vi "UHR-Fleezers Control (host) - Lorentz v3.vi"() -> ()   [LabVIEW 2014] (continued)
                            n445 = Not(x=w776) -> (.not. x?=w775:bool)
                            n446 = Compound Arithmetic op=OR(w779, "Cancel dwell", w775) -> (w778:bool)
                            n447 = node-c288() -> ()  [unwired: 1 in, 1 out]
                            n448 = Select(t=FALSE, s="Pause dwell", f=w778) -> (s? t:f=w781:bool)
                            n449 = Or(x=w781, y=w773) -> (x .or. y?=w774:bool)
                            "Dwell Time (s)" <- w772
                          }
                          n450 = node-c288(w770) -> ()  [unwired: 1 out]
                        }
                      }
                    }
                  }
                }
                frame #4 {
                  n451 = local read "Dip for Protein"() -> (w791:bool)
                  n452 = local read "Dump Beads"() -> (w788:bool)
                  n453 = local write "Cancel dwell"(FALSE ("Cancel dwell")) -> ()
                  n454 = Not(x=w791) -> (.not. x?=w792:bool)
                  n455 = Not(x="Cont. Repeat Dipping?") -> (.not. x?=w794:bool)
                  n456 = Compound Arithmetic op=OR(w792, w794, w788) -> (w790:bool)
                }
              }
            }
          }
        }
      }
      event "Profile": Value Change {
        n457 = event-data() -> ()  [unwired: 1 in, 5 out]
        n458 = flat-sequence {
          tunnel: w803 -> [w806]
          tunnel: w802 -> [w814]
          tunnel: [w808] -> w801
          tunnel: [w807] -> w800
          tunnel: [w805] -> w798
          tunnel: [w804] -> w795
          tunnel: w801 -> [w821]
          tunnel: w800 -> [w820]
          tunnel: [w818] -> w799
          tunnel: w798 -> [w819]
          tunnel: [w817] -> w797
          tunnel: [w816] -> w796
          tunnel: w795 -> [w816]
          tunnel: w799 -> [w825]
          tunnel: w797 -> [w824]
          tunnel: w796 -> [w823]
          frame #0 {
            n459 = call "Read Stage Position.vi"("error in"=w814, "VISA resource name in"=w806) -> ("Current Position"=w804:cluster{dbl, dbl, dbl}, "error out"=w807:errorcluster, "VISA resource name out"=w805:refnum<visa-resource-name>)  [unwired: 1 out]
            "Current Position" <- w804
            n460 = local write "Stage Control Serial Error"(w807) -> ()
            n461 = Unbundle(w804) -> (w811:dbl, w813:dbl, w809:dbl)
            n462 = Add(x=w813, y="Y change (mm)") -> (x+y=w810:dbl)
            n463 = Bundle(w811, w810, w809) -> (w808:cluster{dbl, dbl, dbl})  [unwired: 1 in]
          }
          frame #1 {
            # "move to new position and start saving"
            n464 = local write "Stage Moving"(TRUE ("Stage Moving")) -> ()
            n465 = local write "Start Saving"(TRUE ("Start Saving")) -> ()
            n466 = call "Set Stage Position.vi"("Position"=w821, "error in"=w820, "VISA resource name in"=w819) -> ("error out"=w817:errorcluster, "VISA resource name out"=w818:refnum<visa-resource-name>)  [unwired: 1 out]
          }
          frame #2 {
            # "go back to start"
            n467 = call "Set Stage Position.vi"("Position"=w823, "error in"=w824, "VISA resource name in"=w825) -> ()  [unwired: 3 out]
          }
          frame #3 {
            # "stop saving"
            n468 = local write "Stop Saving"(TRUE ("Stop Saving")) -> ()
            n469 = local write "Stage Moving"(FALSE ("Stage Moving")) -> ()
          }
        }
      }
      event "Move to Position 1", "Move to Position 2", "Move to Position 3", "Move to Position 4", "Move to Position 5", "Lower Ch. Cap.", "Move to Position 6": Value Change {
        n470 = event-data() -> ()  [unwired: 1 in, 5 out]
        n471 = Or(x="Move to Position 5", y="Lower Ch. Cap.") -> (x .or. y?=w832:bool)
        n472 = Build Array("Move to Position 1", "Move to Position 2", "Move to Position 3", "Move to Position 4", w832, "Move to Position 6") -> (w835:bool[])
        n473 = Boolean Array To Number(Boolean array=w835) -> (number=w834:u32)
        n474 = Logarithm Base 2(1:w834) -> (0:w833:dbl)
        n475 = flat-sequence {
          tunnel: w833 -> [w844]
          tunnel: w830 -> [w842]
          tunnel: w829 -> [w841]
          frame #0 {
            n476 = local read "Saved Stage Positions"() -> (w852:dbl[][])
            n477 = Array Subset(array=w852, index (row)=w844, length (row)=1 ("length"), index (col)=1 ("index"), length (col)=3 ("length")) -> (w849:dbl[][])
            n478 = Reshape Array(w849, 3 ("dimension size")) -> (w847:dbl[])
            n479 = Array To Cluster(array=w847) -> (cluster=w846:cluster{"[0]":dbl, "[1]":dbl, "[2]":dbl})
            n480 = call "Set Stage Position.vi"("Position"=w846, "error in"=w841, "VISA resource name in"=w842) -> ("error out"=w845:errorcluster)  [unwired: 2 out]
            n481 = local write "Stage Moving"(TRUE ("Stage Moving")) -> ()
            n482 = local write "Stage Control Serial Error"(w845) -> ()
          }
          frame #1 {
            n483 = local write "Stage Moving"(FALSE ("Stage Moving")) -> ()
            n484 = call <vilib>:"Beep.vi"() -> ()  [unwired: 3 in, 9 out]
          }
        }
      }
      event "Got Bead 1": Value Change {
        n485 = event-data() -> ()  [unwired: 1 in, 5 out]
        n486 = flat-sequence {
          tunnel: w855 -> [w857]
          tunnel: w855 -> [w861]
          frame #0 {
            n487 = for {
              N: w857 -> [_]
              n488 = property on="Pressure Up" class="Bool (strict)"("Val(Sgnl)"=TRUE) -> ()  [unwired: 2 in, 2 out]
            }
          }
          frame #1 {
          }
          frame #2 {
            n489 = Wait (ms)(milliseconds to wait=u32 1000) -> ()  [unwired: 1 out]
          }
          frame #3 {
          }
          frame #4 {
            n490 = Multiply(x=w861, y=2) -> (x*y=w860:i32)
            n491 = for {
              N: w860 -> [_]
              n492 = property on="Vent pressure" class="Bool (strict)"("Val(Sgnl)"=TRUE) -> ()  [unwired: 2 in, 2 out]
            }
          }
          frame #5 {
            n493 = for {
              N: "Number of Pulses for bead 2" -> [_]
              n494 = property on="Pressure Up" class="Bool (strict)"("Val(Sgnl)"=TRUE) -> ()  [unwired: 2 in, 2 out]
            }
          }
        }
        n495 = local read "Number of pulses For laminar flow"() -> (w855:i32)
      }
      event "Force FB Data\nScript": Value Change {
        n496 = event-data() -> ()  [unwired: 1 in, 5 out]
        n497 = flat-sequence {
          tunnel: w871 -> [w875]
          tunnel: w872 -> [w876]
          tunnel: [w876] -> w867
          tunnel: [w875] -> w866
          tunnel: w867 -> [w879]
          tunnel: w866 -> [w878]
          tunnel: ["Trap Trig Fl."] -> w868
          tunnel: [w904] -> w869
          tunnel: w868 -> [w904]
          tunnel: [w908] -> w870
          tunnel: w869 -> [w908]
          tunnel: w870 -> [w910]
          frame #0 {
            n498 = property on="Trap Delta (MHz)" class="DigNum (strict)"("Val(Sgnl)"="Trap Delta Before Moving") -> ()  [unwired: 2 in, 2 out]
          }
          frame #1 {
            n499 = local read "Saved Stage Positions"() -> (w881:dbl[][])
            n500 = property on="Trap Pos. FB Offset Factor" class="DigNum (strict)"("Val(Sgnl)"=i64 0 ("Value (Signaling)")) -> ()  [unwired: 2 in, 2 out]
            n501 = local write "FB Trap Pos Offset"(0.0 ("FB Trap Pos Offset")) -> ()
            n502 = local write "Stage Moving"(TRUE ("Stage Moving")) -> ()
            n503 = call "move to saved stage position.vi"("error in"=w878, "Stage VISA resource name in"=w879, "Position"="Stage Position To Establish FB", "Saved Stage Positions"=w881) -> ("error out"=w877:errorcluster)  [unwired: 1 out]
            n504 = local write "Stage Control Serial Error"(w877) -> ()
          }
          frame #2 {
            n505 = call <vilib>:"Beep.vi"() -> ()  [unwired: 3 in, 9 out]
            n506 = Multiply(x="Wait (s)", y=u32 1000 ("milliseconds to wait")) -> (x*y=w888:u32)
            n507 = property on="Trap Delta (MHz)" class="DigNum (strict)"("Val(Sgnl)"="Starting \nTrap Delta (MHz)") -> ()  [unwired: 2 in, 2 out]
            n508 = local write "Stage Moving"(FALSE ("Stage Moving")) -> ()
            n509 = Wait (ms)(milliseconds to wait=w888) -> ()  [unwired: 1 out]
            n510 = property on="Tab Control 2" class="TabCtl (strict)"("Val(Sgnl)"=T11."Feedback on Trap Position" ("Value (Signaling)")) -> ()  [unwired: 2 in, 2 out]
            n511 = property on="Tab Control" class="TabCtl (strict)"("Val(Sgnl)"=T41."Trap Control (RF)" ("Value (Signaling)")) -> ()  [unwired: 2 in, 2 out]
          }
          frame #3 {
            n512 = property on="Set Reading to\nSetpoint" class="Bool (strict)"("Val(Sgnl)"=TRUE ("Value (Signaling)")) -> ()  [unwired: 2 in, 2 out]
            n513 = Wait (ms)(milliseconds to wait=u32 500) -> ()  [unwired: 1 out]
          }
          frame #4 {
            n514 = property on="Trap Pos. FB ON" class="Bool (strict)"("Val(Sgnl)"=TRUE ("Value (Signaling)")) -> ()  [unwired: 2 in, 2 out]
            n515 = Wait (ms)(milliseconds to wait=u32 250) -> ()  [unwired: 1 out]
          }
          frame #5 {
            n516 = case shown="False" "Trap Trig Fl." {
              frame False {
                n517 = case shown="True" "Green ON after FB ON?" {
                  selector: "Green ON after FB ON?" -> [_ w903]
                  frame False {
                  }
                  frame True {
                    n518 = property on="Green Laser ON" class="Bool (strict)"("Val(Sgnl)"=w903) -> ()  [unwired: 2 in, 2 out]
                  }
                }
              }
              frame True {
              }
            }
            n519 = case shown="True" "Remove Action Offset" {
              tunnel: TRUE ("Value (Signaling)") -> [w900 w901]
              frame False {
                n520 = property on="Remove Unwinding Offset" class="Bool (strict)"("Val(Sgnl)"=w900) -> ()  [unwired: 2 in, 2 out]
              }
              frame True {
                n521 = property on="Remove Action Offset" class="Bool (strict)"("Val(Sgnl)"=w901) -> ()  [unwired: 2 in, 2 out]
              }
            }
            n522 = Wait (ms)(milliseconds to wait=u32 250) -> ()  [unwired: 1 out]
          }
          frame #6 {
            n523 = property on="Start Saving" class="Bool (strict)"("Val(Sgnl)"=TRUE ("Value (Signaling)")) -> ()  [unwired: 2 in, 2 out]
            n524 = Wait (ms)(milliseconds to wait=u32 5000) -> ()  [unwired: 1 out]
          }
          frame #7 {
            w907 = TRUE ("Value (Signaling)")
            n525 = property on="Rem fb disp offset" class="Bool (strict)"("Val(Sgnl)"=w907) -> ()  [unwired: 2 in, 2 out]
            n526 = property on="Remove Offset" class="Bool (strict)"("Val(Sgnl)"=w907) -> ()  [unwired: 2 in, 2 out]
            n527 = Wait (ms)(milliseconds to wait=u32 100) -> ()  [unwired: 1 out]
          }
          frame #8 {
            n528 = case shown="True" w910 {
              frame False {
              }
              frame True {
                n529 = local write "Trap Trig. Fl."(TRUE ("Value (Signaling)")) -> ()
              }
            }
          }
          frame #9 {
            n530 = case shown="True" "Start dipping after?" {
              frame False {
              }
              frame True {
                n531 = flat-sequence {
                  frame #0 {
                    n532 = Multiply(x="Delay before dipping (s)", y=1000.0) -> (x*y=w914:dbl)
                    n533 = Wait (ms)(milliseconds to wait=w914) -> ()  [unwired: 1 out]
                  }
                  frame #1 {
                    n534 = property on="Dip for Protein" class="Bool (strict)"("Val(Sgnl)"=TRUE ("Value (Signaling)")) -> ()  [unwired: 2 in, 2 out]
                    n535 = local write "Scripts"(T2."Dipping" ("Scripts")) -> ()
                  }
                }
              }
            }
          }
        }
      }
      event "Fixed Traps Data\nScript": Value Change {
        n536 = event-data() -> ()  [unwired: 1 in, 5 out]
        n537 = flat-sequence {
          frame #0 {
            n538 = case shown="True" "Green ON" {
              frame False {
              }
              frame True {
                n539 = property on="Green Laser ON" class="Bool (strict)"("Val(Sgnl)"=TRUE) -> ()  [unwired: 2 in, 2 out]
              }
            }
            n540 = local write "Offset (nm)"(0.0 ("Offset (nm)")) -> ()
            n541 = property on="Sample Channel\nFlow" class="Bool (strict)"("Val(Sgnl)"=FALSE ("Value (Signaling)")) -> ()  [unwired: 2 in, 2 out]
            n542 = property on="Trap Delta (MHz)" class="DigNum (strict)"("Val(Sgnl)"="Fixed Traps Trap Delta (MHz)") -> ()  [unwired: 2 in, 2 out]
          }
          frame #1 {
            n543 = Wait (ms)(milliseconds to wait=u32 1000) -> ()  [unwired: 1 out]
          }
          frame #2 {
            n544 = local write "Start Saving"(TRUE ("Start Saving")) -> ()
          }
          frame #3 {
            n545 = local read "Bead Sep. Int. Time (s)"() -> (w925:dbl)
            n546 = Multiply(x=w925, y=1000.0) -> (x*y=w927:dbl)
            n547 = Wait (ms)(milliseconds to wait=w927) -> ()  [unwired: 1 out]
          }
          frame #4 {
            n548 = property on="Remove Offset" class="Bool (strict)"("Val(Sgnl)"=TRUE ("Value (Signaling)")) -> ()  [unwired: 2 in, 2 out]
          }
          frame #5 {
            n549 = property on="Dip for Protein" class="Bool (strict)"("Val(Sgnl)"="Start dipping after?") -> ()  [unwired: 2 in, 2 out]
          }
        }
      }
      event "Got Bead 2": Value Change {
        # "Got A Dig bead and Got DNA bead events changes by Ronen to Got bead 1 and Got bead 2, and modified to enable operation of the thorlabs motors."
        n550 = event-data() -> ()  [unwired: 1 in, 5 out]
        n551 = flat-sequence {
          tunnel: w930 -> [w933]
          frame #0 {
            n552 = case shown="True" "Lumicks Flow During Calibration" {
              tunnel: w933 -> [_ w934]
              frame False {
              }
              frame True {
                n553 = for {
                  N: w934 -> [_]
                  n554 = property on="Pressure Up" class="Bool (strict)"("Val(Sgnl)"=TRUE) -> ()  [unwired: 2 in, 2 out]
                }
              }
            }
          }
          frame #1 {
          }
          frame #2 {
            n555 = Wait (ms)(milliseconds to wait=u32 1000) -> ()  [unwired: 1 out]
          }
          frame #3 {
          }
          frame #4 {
            n556 = case shown="True" "Calibrate after bead 2?" {
              frame False {
              }
              frame True {
                n557 = property on="Cal/Data Acq. Spot" class="Bool (strict)"("Val(Sgnl)"=TRUE) -> ()  [unwired: 2 in, 2 out]
              }
            }
          }
        }
        n558 = local read "Number of pulses For laminar flow"() -> (w930:i32)
      }
      event "Get New Beads": Value Change {
        # "Flow Control determines how many pressure increases are given when moving."
        n559 = event-data() -> ()  [unwired: 1 in, 6 out]
        n560 = flat-sequence {
          tunnel: w939 -> [w941]
          tunnel: w939 -> [w945]
          frame #0 {
            n561 = for {
              N: w941 -> [_]
              n562 = property on="Pressure Up" class="Bool (strict)"("Val(Sgnl)"=TRUE) -> ()  [unwired: 2 in, 2 out]
            }
          }
          frame #1 {
          }
          frame #2 {
            n563 = Wait (ms)(milliseconds to wait=u32 1000) -> ()  [unwired: 1 out]
          }
          frame #3 {
          }
          frame #4 {
            n564 = Multiply(x=2, y=w945) -> (x*y=w944:i32)
            n565 = for {
              N: w944 -> [_]
              n566 = property on="Vent pressure" class="Bool (strict)"("Val(Sgnl)"=TRUE) -> ()  [unwired: 2 in, 2 out]
            }
          }
          frame #5 {
            n567 = for {
              N: "Number of pulses for Bead 1" -> [_]
              n568 = property on="Pressure Up" class="Bool (strict)"("Val(Sgnl)"=TRUE) -> ()  [unwired: 2 in, 2 out]
            }
          }
        }
        n569 = local read "Number of pulses For laminar flow"() -> (w939:i32)
      }
      event "Take Stepping Data": Value Change {
        n570 = event-data() -> ()  [unwired: 1 in, 5 out]
        n571 = local read "Save ave N"() -> (w958:dbl)
        n572 = flat-sequence {
          tunnel: w958 -> [w960]
          tunnel: [w960] -> w953
          tunnel: [w962] -> w954
          tunnel: w953 -> [w962]
          tunnel: [w964] -> w955
          tunnel: w954 -> [w964]
          tunnel: [w967] -> w956
          tunnel: w955 -> [w967]
          tunnel: [w969] -> w957
          tunnel: w956 -> [w969]
          tunnel: [w971] -> w951
          tunnel: w957 -> [w971]
          tunnel: w951 -> [w974]
          tunnel: [w974] -> w950
          tunnel: w950 -> [w975]
          tunnel: [w975] -> w952
          tunnel: w952 -> [w981]
          frame #0 {
            n573 = property on="Save ave N" class="DigNum (strict)"("Val(Sgnl)"="Save ave factor") -> ()  [unwired: 2 in, 2 out]
          }
          frame #1 {
            n574 = Wait (ms)(milliseconds to wait=u32 100) -> ()  [unwired: 1 out]
          }
          frame #2 {
            n575 = local read "Offset 2 Start (MHz)"() -> (w966:dbl)
            n576 = property on="Saved AOD Raster Scan Parameter Sets" class="Arr (strict)"("Index Values"=u32[] [2]) -> ()  [unwired: 2 in, 2 out]
            n577 = property on="Trap Delta (MHz)" class="DigNum (strict)"("Val(Sgnl)"=w966) -> ()  [unwired: 2 in, 2 out]
          }
          frame #3 {
            n578 = property on="Load parameters" class="Bool (strict)"("Val(Sgnl)"=TRUE ("Value (Signaling)")) -> ()  [unwired: 2 in, 2 out]
          }
          frame #4 {
            n579 = Wait (ms)(milliseconds to wait=u32 100) -> ()  [unwired: 1 out]
          }
          frame #5 {
            n580 = property on="Trap Raster Scan" class="Bool (strict)"("Val(Sgnl)"=TRUE ("Value (Signaling)")) -> ()  [unwired: 2 in, 2 out]
          }
          frame #6 {
            n581 = Wait (ms)(milliseconds to wait=u32 1000) -> ()  [unwired: 1 out]
          }
          frame #7 {
            n582 = while {
              stop <- w978 stop-if-true
              n583 = local read "Raster Scanning..."() -> (w980:bool)
              n584 = local read "Saving..."() -> (w979:bool)
              n585 = Not(x=w979) -> (.not. x?=w976:bool)
              n586 = Not(x=w980) -> (.not. x?=w977:bool)
              n587 = And(x=w977, y=w976) -> (x .and. y?=w978:bool)
            }
          }
          frame #8 {
            n588 = property on="Save ave N" class="DigNum (strict)"("Val(Sgnl)"=w981) -> ()  [unwired: 2 in, 2 out]
          }
        }
      }
      event "Step Size (nm)": Value Change {
        n589 = event-data() -> ()  [unwired: 1 in, 5 out]
        n590 = flat-sequence {
          frame #0 {
            n591 = property on="Saved AOD Raster Scan Parameter Sets" class="Arr (strict)"("Index Values"=u32[] [1]) -> ()  [unwired: 2 in, 2 out]
          }
          frame #1 {
            n592 = Multiply(x="N Steps", y="Step Size (nm)") -> (x*y=w983:dbl)
            n593 = property on="Scan Speed AOD (nm/s) 2" class="DigNum (strict)"("Value"="Step Size (nm)") -> ()  [unwired: 2 in, 2 out]
            n594 = property on="Step Size AOD (nm) 2" class="DigNum (strict)"("Value"="Step Size (nm)") -> ()  [unwired: 2 in, 2 out]
            n595 = property on="Scan Range AOD (nm) 2" class="DigNum (strict)"("Value"=w983) -> ()  [unwired: 2 in, 2 out]
          }
        }
      }
      event "Take Detection Laser\nImage": Value Change {
        n596 = event-data() -> ()  [unwired: 1 in, 5 out]
        n597 = flat-sequence {
          tunnel: [w1011] -> w1001
          tunnel: [w1010] -> w994
          tunnel: [w1009] -> w986
          tunnel: [w1014] -> w1002
          tunnel: w1001 -> [w1014]
          tunnel: [w1013] -> w995
          tunnel: w994 -> [w1013]
          tunnel: [w1012] -> w987
          tunnel: w986 -> [w1012]
          tunnel: [w1018] -> w1003
          tunnel: w1002 -> [w1018]
          tunnel: [w1017] -> w996
          tunnel: w995 -> [w1017]
          tunnel: [w1016] -> w988
          tunnel: w987 -> [w1016]
          tunnel: [w1024] -> w1004
          tunnel: w1003 -> [w1024]
          tunnel: [w1023] -> w997
          tunnel: w996 -> [w1023]
          tunnel: [w1022] -> w989
          tunnel: w988 -> [w1022]
          tunnel: [w1028] -> w1005
          tunnel: w1004 -> [w1028]
          tunnel: [w1027] -> w998
          tunnel: w997 -> [w1027]
          tunnel: [w1026] -> w990
          tunnel: w989 -> [w1026]
          tunnel: [w1032] -> w1006
          tunnel: w1005 -> [w1032]
          tunnel: [w1031] -> w999
          tunnel: w998 -> [w1031]
          tunnel: [w1030] -> w991
          tunnel: w990 -> [w1030]
          tunnel: [w1036] -> w1007
          tunnel: w1006 -> [w1036]
          tunnel: [w1035] -> w1000
          tunnel: w999 -> [w1035]
          tunnel: [w1034] -> w992
          tunnel: w991 -> [w1034]
          tunnel: w1007 -> [w1042]
          tunnel: w1000 -> [w1041]
          tunnel: [w1039] -> w993
          tunnel: w992 -> [w1039]
          tunnel: w993 -> [w1043]
          frame #0 {
            n598 = local read "Laser interlacing mode"() -> (w1010:enum32{"Laser ON", "Laser OFF", "Interlace"})
            n599 = local read "Green FB On/Off"() -> (w1009:bool)
            n600 = local read "Green Laser ON"() -> (w1011:bool)
          }
          frame #1 {
            n601 = property on="Green FB On/Off" class="Bool (strict)"("Val(Sgnl)"=FALSE ("Value (Signaling)")) -> ()  [unwired: 2 in, 2 out]
          }
          frame #2 {
            n602 = property on="Green Laser ON" class="Bool (strict)"("Val(Sgnl)"=TRUE ("Value (Signaling)")) -> ()  [unwired: 2 in, 2 out]
            n603 = property on="Flip Green Filter" class="Bool (strict)"("Val(Sgnl)"=TRUE ("Value (Signaling)")) -> ()  [unwired: 2 in, 2 out]
            n604 = property on="Laser interlacing mode" class="RadioBtnsControl (strict)"("Val(Sgnl)"=enum32{"Laser ON", "Laser OFF", "Interlace"}."Laser ON" ("Value (Signaling)")) -> ()  [unwired: 2 in, 2 out]
          }
          frame #3 {
            n605 = Wait (ms)(milliseconds to wait=u32 500) -> ()  [unwired: 1 out]
          }
          frame #4 {
            n606 = property on="Confocal Image" class="Bool (strict)"("Val(Sgnl)"=TRUE ("Value (Signaling)")) -> ()  [unwired: 2 in, 2 out]
          }
          frame #5 {
            n607 = Wait (ms)(milliseconds to wait=u32 2000) -> ()  [unwired: 1 out]
          }
          frame #6 {
            n608 = while {
              stop <- w1037 stop-if-true
              n609 = local read "Saving..."() -> (w1038:bool)
              n610 = Not(x=w1038) -> (.not. x?=w1037:bool)
            }
          }
          frame #7 {
            n611 = property on="Flip Green Filter" class="Bool (strict)"("Val(Sgnl)"=TRUE ("Value (Signaling)")) -> ()  [unwired: 2 in, 2 out]
            n612 = property on="Green Laser ON" class="Bool (strict)"("Val(Sgnl)"=w1042) -> ()  [unwired: 2 in, 2 out]
            n613 = property on="Laser interlacing mode" class="RadioBtnsControl (strict)"("Val(Sgnl)"=w1041) -> ()  [unwired: 2 in, 2 out]
          }
          frame #8 {
            n614 = property on="Green FB On/Off" class="Bool (strict)"("Val(Sgnl)"=w1043) -> ()  [unwired: 2 in, 2 out]
          }
        }
      }
      event "Move in a Circle": Value Change {
        w1045 = dbl[] []
        # "converting distance (d) to angle (a)\na=arcsin(d/2r)"
        # "radius"
        # "radius"
        # "T1 Y"
        # "T1 X"
        n615 = event-data() -> ()  [unwired: 1 in, 5 out]
        n616 = local read "BD 1 Frequency 1 (MHz)"() -> (w1053:dbl)
        n617 = local read "BD 2 Frequency 1 (MHz)"() -> (w1052:dbl)
        n618 = local read "BD 1 Frequency 2 (MHz)"() -> (w1051:dbl)
        n619 = local read "BD 2 Frequency 2 (MHz)"() -> (w1050:dbl)
        n620 = Subtract(x=w1052, y="Center Y Frequency (MHz)") -> (x-y=w1057:dbl)
        n621 = Absolute Value(x=w1057) -> (abs(x)=w1048:dbl)
        n622 = flat-sequence {
          tunnel: w1048 -> [w1060]
          tunnel: [w1060] -> w1047
          frame #0 {
            n623 = local write "Radius (MHz)"(w1060) -> ()
          }
        }
        n624 = node-c288("Time step (ms)") -> (w1059:T37)  [unwired: 3 in]
        n625 = timed-loop {
          timing: w1059 -> [_]
          timing-out: [_] -> w1058
          tunnel: w1053 -> [w1151]
          tunnel: w1052 -> [_]
          tunnel: w1051 -> [w1155]
          tunnel: w1050 -> [_]
          tunnel: "Center Y Frequency (MHz)" -> [w1144]
          shift-right: [w1105] -> _
          shift-left: w1045 -> [w1112]
          shift-right: [w1103] -> _
          shift-left: w1045 -> [w1111]
          shift-right: [w1096] -> _
          shift-left: w1045 -> [w1109]
          shift-right: [w1094] -> _
          shift-left: w1045 -> [w1108]
          tunnel: "Move in a Circle" -> [_]
          tunnel: ["Back to start on finish?"] -> w1049
          tunnel: w1047 -> [_]
          tunnel: w1046 -> [w1126]
          tunnel: w1045 -> [w1107]
          shift-right: [w1078] -> _
          shift-left: 0.0 -> [w1076]
          i -> [w1085]
          stop <- w1149 stop-if-true
          w1093 = 0 ("index")
          w1114 = 1 ("dimension size")
          # "Keep phase within\n2pi so errors don't \nbuild"
          # "Accumulated\nphase"
          # "Current phase"
          # "Trap 2"
          # "Trap 1"
          # "ignore if N = 0"
          # "r"
          # "r"
          # "r"
          # "r"
          # "\"omega*t\""
          # "Trap 2"
          # "Trap separation (radians)"
          # "Trap 1"
          # "Offset (starts\n at bottom of\n the circle)"
          # "omega"
          n626 = node-c288() -> (w1162:i64)  [unwired: 1 in]
          n627 = Divide(x=w1162, y=1000) -> (x/y=w1081:dbl)
          n628 = Divide(x="2D Motion Trap Separation (MHz)", y="Radius (MHz)") -> (x/y=w1136:dbl)
          n629 = Negate(x=w1081) -> (-x=w1080:dbl)
          n630 = Divide(x="Trap 2 phase shift (deg)", y=360.0) -> (x/y=w1127:dbl)
          n631 = Inverse Sine(1:w1136) -> (0:w1072:dbl)
          n632 = Multiply(x=6.283185307179586, y=w1127) -> (x*y=w1073:dbl)
          n633 = Multiply(x=6.283185307179586, y="2D Motion Frequency (Hz)") -> (x*y=w1084:dbl)
          n634 = Select(t=w1081, s="Counterclockwise/Clockwise", f=w1080) -> (s? t:f=w1083:dbl)
          n635 = Multiply(x=w1084, y=w1083) -> (x*y=w1074:dbl)
          n636 = Select(t=w1072, s="Trap shift\nmethod", f=w1073) -> (s? t:f=w1071:dbl)
          n637 = Add(x=w1074, y=w1076) -> (x+y=w1077:dbl)
          n638 = Add(x=w1077, y=w1071) -> (x+y=w1133:dbl)
          n639 = Add(x=w1077, y=1.5707963267948966) -> (x+y=w1082:dbl)
          n640 = Add(x=w1133, y=1.5707963267948966) -> (x+y=w1146:dbl)
          n641 = Cosine(x=w1082) -> (cos(x)=w1160:dbl)
          n642 = Sine(x=w1082) -> (sin(x)=w1159:dbl)
          n643 = Multiply(x=w1160, y="Radius (MHz)") -> (x*y=w1153:dbl)
          n644 = Cosine(x=w1146) -> (cos(x)=w1158:dbl)
          n645 = Sine(x=w1146) -> (sin(x)=w1157:dbl)
          n646 = Multiply(x=w1159, y="Radius (MHz)") -> (x*y=w1152:dbl)
          n647 = Multiply(x=w1158, y="Radius (MHz)") -> (x*y=w1156:dbl)
          n648 = Multiply(x=w1157, y="Radius (MHz)") -> (x*y=w1154:dbl)
          n649 = Add(x=w1153, y=w1151) -> (x+y=w1102:dbl)
          n650 = Add(x=w1152, y=w1144) -> (x+y=w1100:dbl)
          n651 = Greater Or Equal?(x=w1085, y="N steps then stop") -> (x >= y?=w1143:bool)
          n652 = Add(x=w1156, y=w1155) -> (x+y=w1091:dbl)
          n653 = Add(x=w1154, y=w1144) -> (x+y=w1089:dbl)
          n654 = Not Equal To 0?(x="N steps then stop") -> (x != 0?=w1139:bool)
          n655 = And(x=w1143, y=w1139) -> (x .and. y?=w1140:bool)
          n656 = local read "Trap 1 sum mean"() -> (w1123:dbl)
          n657 = local read "Stop All"() -> (w1148:bool)
          n658 = local write "BD 1 Frequency 1 (MHz)"(w1102) -> ()
          n659 = local write "BD 2 Frequency 1 (MHz)"(w1100) -> ()
          n660 = local write "BD 1 Frequency 2 (MHz)"(w1091) -> ()
          n661 = local write "BD 2 Frequency 2 (MHz)"(w1089) -> ()
          n662 = Select(t=w1085, s="test", f=w1123) -> (s? t:f=→"Waveform Chart":dbl)
          n663 = Compound Arithmetic op=OR(w1148, "Stop Moving", w1140) -> (w1149:bool)
          n664 = local read "BD 1 Frequency 3 (MHz)"() -> (w1132:dbl)
          n665 = local read "BD 2 Frequency 3 (MHz)"() -> (w1131:dbl)
          n666 = Select(t=w1107, s="Reset graph", f=w1108) -> (s? t:f=w1088:dbl[])
          n667 = Select(t=w1107, s="Reset graph", f=w1109) -> (s? t:f=w1090:dbl[])
          n668 = Select(t=w1107, s="Reset graph", f=w1111) -> (s? t:f=w1099:dbl[])
          n669 = Select(t=w1107, s="Reset graph", f=w1112) -> (s? t:f=w1101:dbl[])
          n670 = Initialize Array(w1089, w1114) -> (w1115:dbl[])
          n671 = Initialize Array(w1100, w1114) -> (w1118:dbl[])
          n672 = Initialize Array(w1091, w1114) -> (w1116:dbl[])
          n673 = Initialize Array(w1102, w1114) -> (w1119:dbl[])
          n674 = local read "Y RF Frequency Limits (MHz)"() -> (w1129:T24)
          n675 = local read "X RF Frequency Limits (MHz)"() -> (w1130:T24)
          n676 = call "set RF board frequency - interlace.vi"("Board 2 Frequency Limits"=w1129, "Board 1 Frequency Limits"=w1130, "FPGA VI Reference In"=w1126, "Board 2 Frequency 3 (MHz)"=w1131, "Board 1 Frequency 3 (MHz)"=w1132, "Board 2 Frequency 2 (MHz)"=w1089, "Board 2 Frequency 1 (MHz)"=w1100, "Board 1 Frequency 2 (MHz)"=w1091, "Board 1 Frequency 1  (MHz)"=w1102) -> ()  [unwired: 1 in, 2 out]
          n677 = Bundle(w1116, w1115) -> (w1087:cluster{dbl[], dbl[]})  [unwired: 1 in]
          n678 = Bundle(w1119, w1118) -> (w1117:cluster{dbl[], dbl[]})  [unwired: 1 in]
          n679 = Build Array (concatenate)(w1102, w1101) -> (w1106:dbl[])
          n680 = Build Array (concatenate)(w1100, w1099) -> (w1104:dbl[])
          n681 = Build Array (concatenate)(w1091, w1090) -> (w1097:dbl[])
          n682 = Build Array (concatenate)(w1089, w1088) -> (w1095:dbl[])
          n683 = Bundle(w1106, w1104) -> (w1086:cluster{dbl[], dbl[]})  [unwired: 1 in]
          n684 = Bundle(w1097, w1095) -> (w1113:cluster{dbl[], dbl[]})  [unwired: 1 in]
          n685 = Build Array(w1117, w1087, w1086, w1113) -> (→"Trap trajectories":cluster{dbl[], dbl[]}[])
          n686 = case "To pause the process" shown="True" "Pause rotation" {
            frame False {
            }
            frame True {
              n687 = while {
                stop <- w1165 stop-if-true
                n688 = local read "Pause rotation"() -> (w1166:bool)
                n689 = Wait (ms)(milliseconds to wait=u32 10) -> ()  [unwired: 1 out]
                n690 = Not(x=w1166) -> (.not. x?=w1165:bool)
              }
            }
          }
          n691 = Decrement(x="N steps to plot") -> (x-1=w1092:i32)
          n692 = Array Subset(array=w1104, index=w1093, length=w1092) -> (w1103:dbl[])
          n693 = Array Subset(array=w1106, index=w1093, length=w1092) -> (w1105:dbl[])
          n694 = Array Subset(array=w1097, index=w1093, length=w1092) -> (w1096:dbl[])
          n695 = Array Subset(array=w1095, index=w1093, length=w1092) -> (w1094:dbl[])
          n696 = Quotient & Remainder(x=w1077, y=6.283185307179586) -> (x-y*floor(x/y)=w1078:dbl)  [unwired: 1 out]
          n697 = node-c288() -> ()  [unwired: 1 in, 1 out]
        }
        n698 = node-c288(w1058) -> ()  [unwired: 1 out]
        n699 = case shown="True" w1049 {
          tunnel: w1053 -> [_ w1064]
          tunnel: w1052 -> [_ w1063]
          tunnel: w1051 -> [_ w1062]
          tunnel: w1050 -> [_ w1061]
          frame False {
          }
          frame True {
            n700 = flat-sequence {
              tunnel: w1064 -> [w1068]
              tunnel: w1063 -> [w1067]
              tunnel: w1062 -> [w1066]
              tunnel: w1061 -> [w1065]
              frame #0 {
                n701 = local write "BD 1 Frequency 1 (MHz)"(w1068) -> ()
                n702 = local write "BD 2 Frequency 1 (MHz)"(w1067) -> ()
                n703 = local write "BD 1 Frequency 2 (MHz)"(w1066) -> ()
                n704 = local write "BD 2 Frequency 2 (MHz)"(w1065) -> ()
              }
              frame #1 {
                n705 = property on="Update all trap values" class="Bool (strict)"("Val(Sgnl)"=TRUE ("Value (Signaling)")) -> ()  [unwired: 2 in, 2 out]
              }
            }
          }
        }
      }
      event "Stop All": Value Change {
        # "Stopping blue laser before shutting off program"
        n706 = event-data() -> ()  [unwired: 1 in, 5 out]
        n707 = local read "Delay (ms)"() -> (w1176:i32)
        n708 = call "serial write macro.vi"("String"="l0", "Delay (ms)"=w1176, "VISA resource name"=w1179) -> ("read buffer"=w1174:string, "error out"=w1175:errorcluster, "VISA resource name out"=w1178:refnum<visa-resource-name>)
        n709 = local write "read blue buffer"(w1174) -> ()
        n710 = local write "Blue Error Out"(w1175) -> ()
        n711 = VISA Close(VISA resource name=w1178) -> ()  [unwired: 1 in, 1 out]
        n712 = local read "Stop All"() -> (w1180:bool)
      }
      event "Sensitivity", "Offset Current Sign", "Offset Current Value", "Offset Current", "Bias Voltage", "Bias Voltage (mV)", "Filter Type", "Lowpass 3dB Point", "Highpass 3dB Point", "Filter Reset", "Invert Signal", "Gain Mode", "Send Command": Value Change {
        w1187 = 250 ("Delay (ms)")
        n713 = event-data() -> ()  [unwired: 1 in, 5 out]
        n714 = event shown="[0] \"Sensitivity\": Value Change" {
          selector: _ -> [_ _ _ _ _ _ _ _ _ _ _ _ _]
          dyn-events: _ -> [_ _ _ _ _ _ _ _ _ _ _ _ _]
          timeout: _ -> [_ _ _ _ _ _ _ _ _ _ _ _ _]
          tunnel: [w1199 w1207 w1215 w1224 w1234 w1242 w1245 w1249 w1252 w1255 w1258 w1265 "Command"] -> w1186
          tunnel: [w1194 w1201 w1211 w1218 w1228 w1238 _ _ _ _ _ w1261 _] -> w1181
          event "Sensitivity": Value Change {
            n715 = event-data() -> ()  [unwired: 1 in, 5 out]
            n716 = property on="Sensitivity" class="CmbBox"() -> ("Value"=→"Gain":string)  [unwired: 2 in, 2 out]
            n717 = Concatenate Strings("SENS ", "Sensitivity") -> (w1199:string)
            n718 = local read "Gain"() -> (w1196:string)
            n719 = Concatenate Strings("gain set at ", w1196) -> (w1194:string)
          }
          event "Offset Current Sign": Value Change {
            n720 = event-data() -> ()  [unwired: 1 in, 4 out]
            n721 = Boolean To (0,1)(Boolean="Offset Current Sign") -> (0, 1=w1210:i16)
            n722 = Select(t="positive", s="Offset Current Sign", f="negative") -> (s? t:f=w1202:string)
            n723 = Number To Decimal String(number=w1210) -> (decimal integer string=w1209:string)  [unwired: 1 in]
            n724 = Concatenate Strings("IOSN " ("string"), w1209) -> (w1207:string)
            n725 = Concatenate Strings("offset current sign ", w1202) -> (w1201:string)
          }
          event "Offset Current Value": Value Change {
            n726 = event-data() -> ()  [unwired: 1 in, 5 out]
            n727 = property on="Offset Current Value" class="CmbBox"() -> ("Value"=→"Read offset current":string)  [unwired: 2 in, 2 out]
            n728 = local read "Read offset current"() -> (w1212:string)
            n729 = Concatenate Strings("IOLV ", "Offset Current Value") -> (w1215:string)
            n730 = Concatenate Strings("offset current value ", w1212) -> (w1211:string)
          }
          event "Offset Current": Value Change {
            n731 = event-data() -> ()  [unwired: 1 in, 5 out]
            n732 = Boolean To (0,1)(Boolean="Offset Current") -> (0, 1=w1227:i16)
            n733 = Select(t="on", s="Offset Current", f="off") -> (s? t:f=w1219:string)
            n734 = Number To Decimal String(number=w1227) -> (decimal integer string=w1226:string)  [unwired: 1 in]
            n735 = Concatenate Strings("IOON " ("string"), w1226) -> (w1224:string)
            n736 = Concatenate Strings("offset current ", w1219) -> (w1218:string)
          }
          event "Bias Voltage": Value Change {
            n737 = event-data() -> ()  [unwired: 1 in, 5 out]
            n738 = Boolean To (0,1)(Boolean="Bias Voltage") -> (0, 1=w1235:i16)
            n739 = Number To Decimal String(number=w1235) -> (decimal integer string=w1236:string)  [unwired: 1 in]
            n740 = Select(t="on", s="Bias Voltage", f="off") -> (s? t:f=w1229:string)
            n741 = Concatenate Strings("BSON " ("string"), w1236) -> (w1234:string)
            n742 = Concatenate Strings("bias voltage", w1229) -> (w1228:string)
          }
          event "Bias Voltage (mV)": Value Change {
            n743 = event-data() -> ()  [unwired: 1 in, 5 out]
            n744 = Number To Decimal String(number="Bias Voltage (mV)") -> (decimal integer string=w1244:string)  [unwired: 1 in]
            n745 = Number To Fractional String(number="Bias Voltage (mV)") -> (F-format string=w1239:string)  [unwired: 3 in]
            n746 = Concatenate Strings("BSLV " ("string"), w1244) -> (w1242:string)
            n747 = Concatenate Strings("bias voltage value ", w1239) -> (w1238:string)
          }
          event "Filter Type": Value Change {
            n748 = event-data() -> ()  [unwired: 1 in, 5 out]
            n749 = Concatenate Strings("FLTT " ("string"), "Filter Type") -> (w1245:string)
          }
          event "Lowpass 3dB Point": Value Change {
            n750 = event-data() -> ()  [unwired: 1 in, 5 out]
            n751 = Concatenate Strings("LFRQ " ("string"), "Lowpass 3dB Point") -> (w1249:string)
          }
          event "Highpass 3dB Point": Value Change {
            n752 = event-data() -> ()  [unwired: 1 in, 5 out]
            n753 = Concatenate Strings("HFRQ " ("string"), "Highpass 3dB Point") -> (w1252:string)
          }
          event "Filter Reset": Value Change {
            n754 = event-data() -> ()  [unwired: 1 in, 5 out]
            n755 = Select(t="ROLD", s="Filter Reset", f="") -> (s? t:f=w1255:string)
          }
          event "Gain Mode": Value Change {
            n756 = event-data() -> ()  [unwired: 1 in, 5 out]
            n757 = Concatenate Strings("GNMD " ("string"), "Gain Mode") -> (w1258:string)
          }
          event "Invert Signal": Value Change {
            n758 = event-data() -> ()  [unwired: 1 in, 5 out]
            n759 = Boolean To (0,1)(Boolean="Invert Signal") -> (0, 1=w1268:i16)
            n760 = Number To Decimal String(number=w1268) -> (decimal integer string=w1267:string)  [unwired: 1 in]
            n761 = Concatenate Strings("INVT " ("string"), w1267) -> (w1265:string)
            n762 = Select(t="signal inverted", s="Invert Signal", f="signal not inverted") -> (s? t:f=w1261:string)
          }
          event "Send Command": Value Change {
            n763 = event-data() -> ()  [unwired: 1 in, 5 out]
          }
        }
        "Command Sent" <- w1186
        n764 = local read "Save Event Log?"() -> (w1182:bool)
        n765 = local read "Saving..."() -> (w1183:bool)
        n766 = And(x=w1182, y=w1183) -> (x .and. y?=w1184:bool)
        n767 = case shown="True" w1184 {
          tunnel: w1181 -> [_ w1191]
          frame False {
          }
          frame True {
            n768 = local read "Time (s)"() -> (w1192:dbl)
            n769 = local read "log file ref"() -> (w1193:refnum<file>)
            n770 = call "write to event log.vi"("log file ref"=w1193, "time"=w1192, "input string"=w1191) -> ()  [unwired: 8 in]
          }
        }
        n771 = call "preamp serial write macro.vi"("String"=w1186, "Delay (ms)"=w1187, "VISA resource name"=w1190) -> ("read buffer"=→"Reply":string, "error out"=w1189:errorcluster)  [unwired: 1 out]
        n772 = call "preamp serial write macro.vi"("String"=w1186, "Delay (ms)"=w1187, "VISA resource name"=w1185) -> ()  [unwired: 3 out]
        n773 = local write "Preamp Error Out"(w1189) -> ()
      }
    }
    n774 = node-c288() -> ()  [unwired: 1 in, 1 out]
  }
  n775 = flat-sequence "Safety limits on RF frequencies and amplitudes (for AOM protection)" {
    tunnel: [w1272] -> w20
    tunnel: [w1270] -> w22
    tunnel: [w1273] -> w23
    tunnel: [w1274] -> w21
    tunnel: w4 -> [w1272]
    tunnel: T24 {"Minimum"=0.0, "Maximum"=50.0, "Increment"=1.0} ("Data Entry Limits") -> [w1270]
    tunnel: w9 -> [w1271]
    tunnel: [w1271] -> w24
    frame #0 {
      w1274 = T24 {"Minimum"=0.0, "Maximum"=40.0, "Increment"=0.1} ("Min Max Inc")
      w1273 = T24 {"Minimum"=0.0, "Maximum"=45.0, "Increment"=1.0} ("Data Entry Limits")
      n776 = property on="BD 2 Frequency 1 (MHz)" class="DigNum (strict)"("Data Range"=w1274) -> ()  [unwired: 2 in, 2 out]
      n777 = property on="BD 2 Frequency 3 (MHz)" class="DigNum (strict)"("Data Range"=w1274) -> ()  [unwired: 2 in, 2 out]
      n778 = property on="BD 2 Frequency 2 (MHz)" class="DigNum (strict)"("Data Range"=w1274) -> ()  [unwired: 2 in, 2 out]
      n779 = property on="BD 1 Frequency 1 (MHz)" class="DigNum (strict)"("Data Range"=w1272) -> ()  [unwired: 2 in, 2 out]
      n780 = property on="BD 1 Frequency 2 (MHz)" class="DigNum (strict)"("Data Range"=w1272) -> ()  [unwired: 2 in, 2 out]
      n781 = property on="BD 1 Frequency 3 (MHz)" class="DigNum (strict)"("Data Range"=w1272) -> ()  [unwired: 2 in, 2 out]
      n782 = property on="BD 2 Amplitude 1 (%)" class="DigNum (strict)"("Data Range"=w1273) -> ()  [unwired: 2 in, 2 out]
      n783 = property on="BD 2 Amplitude 2 (%)" class="DigNum (strict)"("Data Range"=w1273) -> ()  [unwired: 2 in, 2 out]
      n784 = property on="BD 2 Amplitude 3 (%)" class="DigNum (strict)"("Data Range"=w1273) -> ()  [unwired: 2 in, 2 out]
      n785 = property on="BD 1 Amplitude 3 (%)" class="DigNum (strict)"("Data Range"=w1270) -> ()  [unwired: 2 in, 2 out]
      n786 = property on="BD 1 Amplitude 2 (%)" class="DigNum (strict)"("Data Range"=w1270) -> ()  [unwired: 2 in, 2 out]
      n787 = property on="BD 1 Amplitude 1 (%)" class="DigNum (strict)"("Data Range"=w1270) -> ()  [unwired: 2 in, 2 out]
      "X RF Frequency Limits (MHz)" <- w1272
      "X RF Amplitude Limits (%)" <- w1270
      "Y RF Amplitude Limits (%)" <- w1273
      "Y RF Frequency Limits (MHz)" <- w1274
    }
  }
  n788 = stacked-sequence "Host initialization sequence - order matters!" {
    tunnel: w24 -> [_ w1294 w1386 _ w1443 w1452 w1519 w1543 _ w1585 _]
    tunnel: [_ _ _ _ _ _ _ _ _ w1585 _] -> w13
    tunnel: [_ _ _ _ _ _ _ _ _ w1584 _] -> w26
    tunnel: w23 -> [_ _ _ _ _ _ w1517 _ _ _ _]
    tunnel: w22 -> [_ _ _ _ _ _ w1516 _ _ _ _]
    tunnel: w21 -> [_ _ _ _ _ _ w1515 _ _ _ _]
    tunnel: w20 -> [_ _ _ _ _ _ w1496 _ _ _ _]
    tunnel: [_ _ _ _ _ _ _ _ w1578 _ _] -> _
    tunnel: [_ _ _ _ _ _ _ _ _ _ w1586] -> w3
    tunnel: [_ _ _ _ _ _ _ _ _ _ w1587] -> w2
    frame #0 {
    }
    frame #1 {
      w1326 = 10.0 ("y")
      w1327 = 32767.0 ("y")
      w1311 = 6.0  # clock mult.
      w1310 = 49152000.0  # TCXO frequ.
      # "Initialize some FPGA settings"
      n789 = local read "Not-Interlacing Set"() -> (w1366:enum32{"Set 1", "Set 2", "Set 3"})
      n790 = local write "Trap Pos FIFO Timeout"(u16 0 ("Trap Pos FIFO Timeout")) -> ()
      n791 = local read "Interlace"() -> (w1364:bool)
      n792 = local read "Desired Scan Incr (V)"() -> (w1338:dbl)
      n793 = local read "BD 1 Delay (ticks)"() -> (w1373:u8)
      n794 = local read "Number Interlace Sets"() -> (w1365:u8)
      n795 = local read "BD 2 Delay (Ticks)"() -> (w1374:u8)
      n796 = property on="AI Count (ticks)" class="DigNum (strict)"("Val(Sgnl)"="AI Count (ticks)") -> ()  [unwired: 2 in, 2 out]
      n797 = local read "AO1"() -> (w1332:dbl)
      n798 = local read "AO2"() -> (w1333:dbl)
      n799 = local read "Next trap write delay (ticks)"() -> (w1375:u8)
      n800 = local read "Number of scans (MCL)"() -> (w1342:u64)
      n801 = local read "Cycles/step (MCL)"() -> (w1341:u64)
      n802 = local read "Scan steps (MCL)"() -> (w1340:u64)
      n803 = local read "Continuous MCL Scanning"() -> (w1343:bool)
      n804 = Multiply(x=w1332, y=w1327) -> (x*y=w1330:dbl)
      n805 = Multiply(x=w1333, y=w1327) -> (x*y=w1328:dbl)
      n806 = Build Array("DIO count 1 (ticks)", "DIO count 2 (ticks)", "DIO count 3 (ticks)") -> (w1359:u16[])
      n807 = local read "Fast Scan Dir"() -> (w1344:bool)
      n808 = local read "2D or 1D Scan"() -> (w1356:bool)
      n809 = local read "N Acq Sets (Traps + Fl.)"() -> (w1352:i16)
      n810 = local read "Scan Increment (MHz)"() -> (w1315:dbl)
      n811 = Divide(x=w1330, y=w1326) -> (x/y=w1331:dbl)
      n812 = Divide(x=w1328, y=w1326) -> (x/y=w1329:dbl)
      n813 = To Unsigned Byte Integer(number=w1366) -> (unsigned 8bit integer=w1361:u8)
      n814 = Split 1D Array(array=w1359, index=w1365) -> (first subarray=w1357:u16[])  [unwired: 1 out]
      n815 = Multiply(x=w1338, y=32767.0) -> (x*y=w1336:dbl)
      n816 = To Word Integer(number=w1331) -> (16bit integer=w1277:i16)
      n817 = To Word Integer(number=w1329) -> (16bit integer=w1276:i16)
      n818 = Index Array(array=w1359, index=w1361) -> (element=w1360:u16)
      n819 = Add Array Elements(numeric array=w1357) -> (sum=w1358:u16)
      n820 = Multiply(x=w1310, y=w1311) -> (x*y=w1312:dbl)
      n821 = Divide(x=w1336, y=10.0) -> (x/y=w1337:dbl)
      n822 = Select(t=w1358, s=w1364, f=w1360) -> (s? t:f=w1367:u16)
      n823 = Not(x=w1344) -> (.not. x?=w1345:bool)
      n824 = To Word Integer(number=w1337) -> (16bit integer=w1339:i16)
      n825 = property on="2D or 1D Scan" class="Bool (strict)"("Val(Sgnl)"=w1356) -> ()  [unwired: 2 in, 2 out]
      n826 = Divide(x=40000000.0, y="AI Count (ticks)") -> (x/y=w1348:dbl)
      n827 = local write "Update Count (MCL)"(w1367) -> ()
      n828 = local write "Total Counts (ticks)"(w1367) -> ()
      n829 = Divide(x=w1348, y="FPGA Ave.") -> (x/y=w1347:dbl)
      n830 = local write "AI rate (Hz)"(w1348) -> ()
      n831 = Multiply(x=w1315, y=1000.0) -> (x*y=w1308:dbl)
      n832 = local write "Ave. Rate (Hz)"(w1347) -> ()
      n833 = Reciprocal(x=w1347) -> (1/x=w1346:dbl)
      n834 = Scale By Power Of 2(n=48, x=w1308) -> (x*2^n=w1307:dbl)
      n835 = local write "Ave. Period (s)"(w1346) -> ()
      n836 = Divide(x=w1307, y=w1312) -> (x/y=w1313:dbl)
      n837 = To Quad Integer(1:w1313) -> (0:w1316:i64)
      n838 = local read "Setpoints (V)"() -> (w1301:cluster{"Set 1":dbl, "Set 2":dbl})
      n839 = local read "# Samples/channel"() -> (w1323:u32)
      n840 = local read "Feedback On/Off"() -> (w1298:cluster{"Set 1":bool, "Set 2":bool})
      n841 = local read "T3 Y (V)"() -> (w1281:dbl)
      n842 = local read "T3 X (V)"() -> (w1280:dbl)
      n843 = local read "Trap intensity output range"() -> (w1291:cluster{"Normal High":i16, "Normal Low":i16})
      n844 = local read "All FB On/Off"() -> (w1297:bool)
      n845 = local read "Number of F/B Scans (AOD)"() -> (w1322:u16)
      n846 = local read "Trap Intensity PID Gains"() -> (w1290:T14)
      n847 = local read "Cycles/step (AOD)"() -> (w1318:u64)
      n848 = local read "Scan steps (AOD)"() -> (w1317:u64)
      n849 = Multiply(x=w1317, y=w1318) -> (x*y=w1319:u64)
      n850 = Multiply(x=w1319, y=u64 2) -> (x*y=w1321:u64)
      n851 = Multiply(x=w1321, y=w1322) -> (x*y=w1324:u64)
      n852 = Multiply(x=3276.7, y=w1301) -> (x*y=w1302:cluster{"Set 1":dbl, "Set 2":dbl})
      n853 = local read "Scan BD"() -> (w1306:bool)
      n854 = Multiply(x=w1281, y=32767.0) -> (x*y=w1287:dbl)
      n855 = And(x=w1298, y=w1297) -> (x .and. y?=w1299:cluster{"Set 1":bool, "Set 2":bool})
      n856 = To Word Integer(number=w1302) -> (16bit integer=w1303:cluster{"Set 1":i16, "Set 2":i16})
      n857 = Multiply(x=w1280, y=32767.0) -> (x*y=w1284:dbl)
      n858 = local read "Sets to FIFO (Traps)"() -> (w1369:T22)
      n859 = Divide(x=w1324, y=w1323) -> (x/y=w1325:dbl)
      n860 = Unbundle By Name(w1299) -> ("Set 1"=w1295:bool, "Set 2"=w1296:bool)
      n861 = Unbundle By Name(w1303) -> ("Set 1"=w1304:i16, "Set 2"=w1305:i16)
      n862 = Divide(x=w1287, y=10.0) -> (x/y=w1288:dbl)
      n863 = Divide(x=w1284, y=10.0) -> (x/y=w1283:dbl)
      n864 = To Unsigned Word Integer(number=w1288) -> (unsigned 16bit integer=w1279:u16)
      n865 = To Unsigned Word Integer(number=w1283) -> (unsigned 16bit integer=w1278:u16)
      n866 = local read "FPGA error out"() -> (w1293:errorcluster)
      n867 = local write "Data points/scan (f/b)"(w1321) -> ()
      n868 = local write "Data points/scans"(w1324) -> ()
      n869 = local write "N sets should be saved"(w1325) -> ()
      n870 = Unbundle By Name(w1369) -> ("Set 1"=w1370:bool, "Set 2"=w1371:bool, "Set 3"=w1372:bool)
      n871 = xnode "Read/Write Control"("FPGA VI Reference In"=w1294, "error in"=w1293, "ai count"="AI Count (ticks)", "Interlace ON/OFF"=w1364, "Number Interlace Cycles"=w1365, "Set 1"=w1370, "Set 2"=w1371, "Set 3"=w1372, "FB On/Off Set 1"=w1295, "FB On/Off Set 2"=w1296, "Interlace Off Parameters"=w1366, "FB Setpoint Set 1"=w1304, "FB Setpoint Set 2"=w1305, "Piezo Trap Y (AO4)"=w1279, "Piezo Trap X (AO5)"=w1278, "FB Gains"=w1290, "FB output range"=w1291, "Cycles per step"=w1318, "Scan BD"=w1306, "Number of scans"=w1322, "Scan steps"=w1317, "Scan freq.  increment"=w1316, "AO1"=w1277, "AO2"=w1276, "Scan freq.  increment (MCL)"=w1339, "Scan steps (MCL)"=w1340, "Cycles per step (MCL)"=w1341, "Number of scans (MCL)"=w1342, "MCL count"=w1367, "Cont. Scan (MCL)"=w1343, "MCL Scan Axis"=w1345, "1D or 2D Scan?"=w1356, "N of AI1 Int Acq Sets"=w1352, "Amp switch delay"="Amp switch delay", "Swap F1 and F2"="Swap F1 and F2", "APD to FIFO"=FALSE, "DIO count 1 (ticks)"="DIO count 1 (ticks)", "DIO count 2 (ticks)"="DIO count 2 (ticks)", "DIO count 3 (ticks)"="DIO count 3 (ticks)", "BD 1 Delay (ticks)"=w1373, "BD 2 Delay (Ticks)"=w1374, "Next trap write delay (ticks)"=w1375) -> ("error out"=w1292:errorcluster)  [unwired: 1 out]
      n872 = local write "FPGA error out"(w1292) -> ()
    }
    frame #2 {
      # "Initialize some more FPGA settings"
      n873 = local read "Trap Pos FB Monitor\nT1 or T2"() -> (w1397:bool)
      n874 = local read "Trap Pos FB Negate Action"() -> (w1398:bool)
      n875 = local read "Trap Pos. FB Offset Factor"() -> (w1399:i64)
      n876 = local read "Trap Pos. FB Mult Factor"() -> (w1400:i64)
      n877 = local read "Trap Pos. AI1 X Pre-scale"() -> (w1402:u16)
      n878 = local read "Trap Pos FB Int Count"() -> (w1404:u16)
      n879 = local read "Green Laser ON"() -> (w1376:bool)
      n880 = local read "Neg. TTrig FPGA"() -> (w1405:bool)
      n881 = local read "Trap Pos. FB Range"() -> (w1381:T18)
      n882 = local read "Trap Pos. FB Gains"() -> (w1382:T17)
      n883 = local read "Dynamic Force FB (ronen)"() -> (w1383:bool)
      n884 = Multiply(x="Green Intensity % (FB OFF)", y=655.35) -> (x*y=w1391:dbl)
      n885 = Multiply(x="Red FB Setpoint (mV)", y=3.2767) -> (x*y=w1413:dbl)
      n886 = Multiply(x="Red Intensity % (FB OFF)", y=655.35) -> (x*y=w1417:dbl)
      n887 = Unbundle By Name("Red FB Gains") -> ("proportional gain (Kc)"=w1422:i16, "integral gain (Kc*Ts/Ti)"=w1423:i16, "derivative gain (Kc*Td/Ts)"=w1424:i16)
      n888 = Multiply(x="Green FB Setpoint (mV)", y=3.2767) -> (x*y=w1394:dbl)
      n889 = To Unsigned Word Integer(number=w1391) -> (unsigned 16bit integer=w1393:u16)
      n890 = To Unsigned Word Integer(number=w1417) -> (unsigned 16bit integer=w1420:u16)
      n891 = To Word Integer(number=w1413) -> (16bit integer=w1416:i16)
      n892 = local read "Differential FB?"() -> (w1407:bool)
      n893 = To Word Integer(number=w1394) -> (16bit integer=w1396:i16)
      n894 = local read "Laser interlacing mode"() -> (w1379:enum32{"Laser ON", "Laser OFF", "Interlace"})
      n895 = local read "Invert laser interlacing"() -> (w1380:bool)
      n896 = Unbundle By Name("Green FB Gains") -> ("proportional gain (Kc)"=w1410:i16, "integral gain (Kc*Ts/Ti)"=w1411:i16, "derivative gain (Kc*Td/Ts)"=w1412:i16)
      n897 = Select(t=w1379, s=w1376, f=enum32{"Laser ON", "Laser OFF", "Interlace"}."Laser OFF" ("Green laser mode")) -> (s? t:f=w1378:enum32{"Laser ON", "Laser OFF", "Interlace"})
      n898 = local read "FPGA error out"() -> (w1384:errorcluster)
